vi "ClearOverload.vi"(0 "device session in":refnum<class "Device Session.lvclass">, 11 "error in":errorcluster) -> (4 "device session out":refnum<class "Device Session.lvclass">, 6 "min wait time (ms)":u32=250000000, 15 "error out":errorcluster)   [LabVIEW 2015, in "Device Session.lvclass"]
doc: "Selects an external clock source and configures the external clock rate. When using an external clock, you must run the <B>Disable Data Clock</B> VI before disconnecting the external clock source.\n\n<B>Input Parameters</B>\n\n<B>device session in</B> is a reference to the session containing sessions to all instrument design libraries used in this sample project. This parameter is obtained from the 'Open Session' VI.\n\n<B>external clock source</B> specifies the source of the external clock.\n\n'Clock In' (default): specifies that the clock source is the Clock In signal from the device front panel.\n'PXIe DStar A': specifies that the clock source is the signal from the PXIe DStar A line.\n\n<B>external clock rate (Hz)</B> specifies the clock rate of the external clock. The default value is 250.\n\n<B>error in</B> describes error conditions that occur before this node runs. This input provides standard 'error in' functionality.\n\n<B>Output Parameters</B>\n\n<B>device session out</B> passes a reference to the session to the next VI.\n\n<B>actual adc clock rate (Hz)</B> returns coerced ADC clock rate in Hz.\n\n<B>error out</B> contains error information. This output provides standard 'error out' functionality."
uses:
  Device Session.lvclass
  Device Session.lvclass/Device Session.ctl
  <instrlib>/HSAI-RIO/Config/Interface/v1/Host/niHSAI Config v1 Host.lvclass
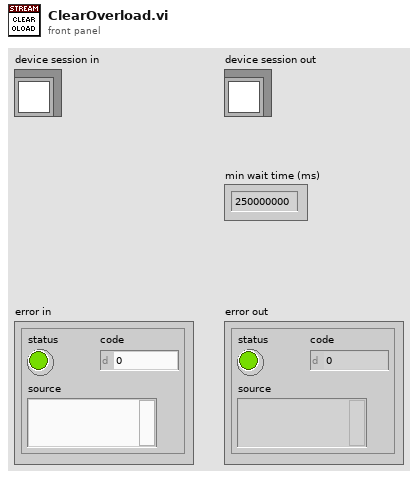
[diagram p1: front panel]
types:
  T1 = typedef "Device Session.lvclass/Device Session Object.ctl" = cluster{"ni5171R FPGA Reference":T2, "niHSAI config":refnum<class "niHSAI Config v1 Host.lvclass">, "configured scaling coefficients":cluster{"gain":dbl, "offset":dbl}[], "number of channels to stream":u8, "selected acq channels":bool[], "number of channels":u32, "actual channel configuration":T3[], "configured channels":bool[], "sample clock rate (Hz)":dbl}
  T2 = typedef "Device Session.lvclass/FPGA Refnum.ctl" = refnum<k20>
  T3 = typedef "niHSAI Types v1 Host.lvlib/Channel Configuration.ctl" = cluster{"channel":u32, "coupling":T4, "impedance":T5, "bandwidth":T6, "vertical range":dbl, "vertical offset":dbl}
  T4 = typedef "niHSAI Types v1 Host.lvlib/Coupling.ctl" = enum8{"Default", "DC", "AC"}
  T5 = typedef "niHSAI Types v1 Host.lvlib/Impedance.ctl" = enum8{"Default", "1 mega ohm", "50 ohm"}
  T6 = typedef "niHSAI Types v1 Host.lvlib/Bandwidth.ctl" = enum8{"Default", "Full Bandwidth", "Anti-alias Filter"}
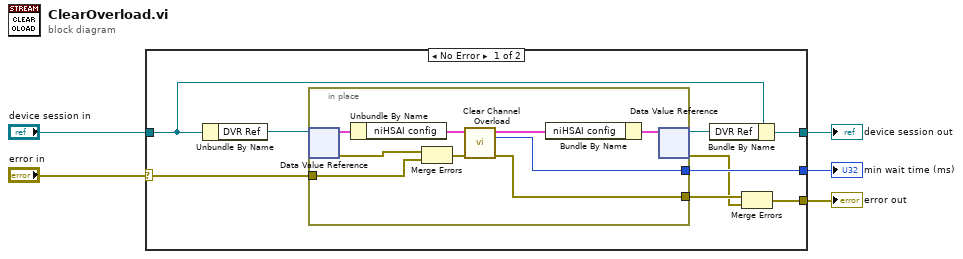
[diagram p0: block diagram]
diagram:
  n1 = case shown="No Error" "error in" {
    selector: "error in" -> [w14 w25]
    tunnel: "device session in" -> [w10 w24]
    tunnel: [w9 w24] -> w3
    tunnel: [w12 w25] -> w2
    tunnel: [w8 _] -> w1
    frame No Error {
      n2 = Unbundle By Name(w10) -> ("DVR Ref"=w11:refnum<data-value>)
      n3 = in-place {
        in-place-border: w14 -> [w15]
        in-place-border: [w18] -> w7
        in-place-border: [w17] -> w8
        n4 = in-place-dvr #1(w11) -> (w22:T1, w16:errorcluster)
        n5 = Unbundle By Name(w22) -> ("niHSAI config"=w21:refnum<class "niHSAI Config v1 Host.lvclass">)
        n6 = Merge Errors(w16, w15) -> (w19:errorcluster)
        n7 = call-dynamic "Clear Channel Overload.vi"("session in"=w21, "error in"=w19) -> ("session out"=w20:refnum<class "niHSAI Config v1 Host.lvclass">, "min wait time (ms)"=w17:u32, "error out"=w18:errorcluster)  [unwired: 11 in]
        n8 = Bundle By Name(cluster=w22, "niHSAI config"=w20) -> (w23:T1)
        n9 = in-place-dvr #1(w23) -> (w13:refnum<data-value>, w6:errorcluster)
      }
      n10 = Bundle By Name(cluster=w10, "DVR Ref"=w13) -> (w9:refnum<class "Device Session.lvclass">)
      n11 = Merge Errors(w7, w6) -> (w12:errorcluster)
    }
    frame Error {
    }
  }
  "error out" <- w2
  "device session out" <- w3
  "min wait time (ms)" <- w1
